vi "UDT_admittanceLibrary_InitialConditions FGV.vi"() -> (3 "Unit Test Framework Results":T1)   [LabVIEW 2017]
doc: "Use this template to create a user-defined test VI. Define your test requirements and wire the results to the <b>Result (Test)</b> control. Do not modify the <b>Unit Test Framework Results</b> indicator."
uses:
  <vilib>/utf/common/utf_test_result_troll.ctl
  <vilib>/utf/common/utf_test_result.ctl
  <vilib>/utf/common/utf_test_result_failure.ctl
  <vilib>/utf/common/utf_test_comparison_operators.ctl
  <vilib>/utf/common/utf_vi_tag.ctl
  RT/Admittance Controller/Controls/initial conditions control.ctl
  <vilib>/Control Software Solutions Ltd/UTF Helper/SubVIs/UTF Double Not Equals.vi
  <vilib>/Control Software Solutions Ltd/UTF Helper/SubVIs/UTF Double Equals.vi
  RT/Admittance Controller/admittanceControllerLibrary.lvlib
  <vilib>/Control Software Solutions Ltd/UTF Helper/Unit Test Helper.lvlib
  <vilib>/utf/NI_UnitTestFramework.lvlib
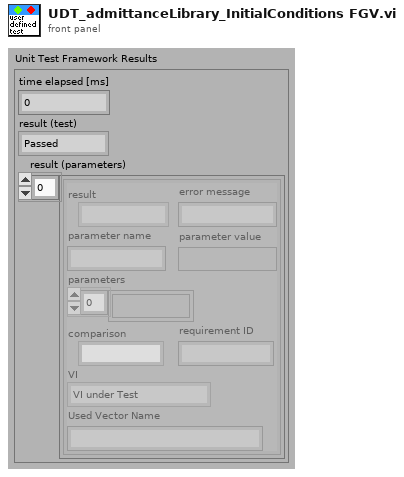
[diagram p1: front panel]
types:
  T1 = typedef "NI_UnitTestFramework.lvlib/utf_test_result_troll.ctl" = cluster{"time elapsed [ms]":u32, "result (test)":T2, "result (parameters)":T3[]}
  T2 = typedef "NI_UnitTestFramework.lvlib/utf_test_result.ctl" = enum16{"Passed", "Failed", "Error", "Skipped", "Not Processed"}
  T3 = typedef "NI_UnitTestFramework.lvlib/utf_test_result_failure.ctl" = cluster{"result":T2, "error message":string, "parameter name":string, "parameter value":variant, "parameters":variant[], "comparison":T4, "requirement ID":string, "VI":T5, "Used Vector Name":string}
  T4 = typedef "NI_UnitTestFramework.lvlib/utf_test_comparison_operators.ctl" = enum16{"=", "!=", ">", ">=", "<", "<=", "range", "symmetric tolerance", "asymmetric tolerance", "string contains", "string not contain", "array size", "string length", "array range", "by element", "array range (limit array)", "user-defined", "array contains", "array not contain", "vector length", "= (elm)", "!= (elm)", "= (case insensitive)", "!= (case insensitive)"}
  T5 = typedef "NI_UnitTestFramework.lvlib/utf_vi_tag.ctl" = enum16{"Setup VI", "VI under Test", "Teardown VI"}
  T6 = typedef "admittanceControllerLibrary.lvlib/initial conditions control.ctl" = enum16{"get", "set"}
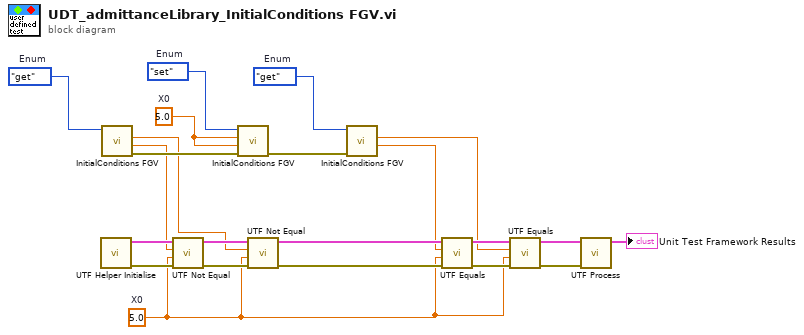
[diagram p0: block diagram]
diagram:
  w3 = 5.0  # X0
  w18 = initial_conditions_control."get"  # Enum
  w20 = initial_conditions_control."get"  # Enum
  w21 = 5.0  # X0
  w22 = initial_conditions_control."set"  # Enum
  n1 = call <vilib>:"UTF Helper Initialise.vi"() -> ("error out"=w14:errorcluster, "results array"=w15:T3[])  [unwired: 10 in]
  n2 = call "InitialConditions FGV.vi"("Enum"=w20) -> ("error out"=w19:errorcluster, "y0"=w11:dbl, "x0"=w10:dbl)  [unwired: 8 in]
  n3 = call-poly <vilib>:"UTF Not Equal.vi"("error in (no error)"=w14, "Test Value"=w3, "Input"=w11, "Input Results"=w15) -> ("error out"=w13:errorcluster, "Output Results"=w12:T3[])  [unwired: 6 in]
  n4 = call "InitialConditions FGV.vi"("error in (no error)"=w19, "Y0"=w21, "X0"=w21, "Enum"=w22) -> ("error out"=w17:errorcluster)  [unwired: 5 in, 2 out]
  n5 = call-poly <vilib>:"UTF Not Equal.vi"("error in (no error)"=w13, "Test Value"=w3, "Input"=w10, "Input Results"=w12) -> ("error out"=w8:errorcluster, "Output Results"=w9:T3[])  [unwired: 6 in]
  n6 = call "InitialConditions FGV.vi"("error in (no error)"=w17, "Enum"=w18) -> ("y0"=w5:dbl, "x0"=w4:dbl)  [unwired: 7 in, 1 out]
  n7 = call-poly <vilib>:"UTF Equals.vi"("error in (no error)"=w8, "Test Value"=w3, "Input"=w5, "Input Results"=w9) -> ("error out"=w6:errorcluster, "Output Results"=w7:T3[])  [unwired: 6 in]
  n8 = call-poly <vilib>:"UTF Equals.vi"("error in (no error)"=w6, "Test Value"=w3, "Input"=w4, "Input Results"=w7) -> ("error out"=w1:errorcluster, "Output Results"=w2:T3[])  [unwired: 6 in]
  n9 = call <vilib>:"UTF Process.vi"("error in (no error)"=w1, "results array"=w2) -> ("Unit Test Framework Results"=→"Unit Test Framework Results":T1)  [unwired: 9 in]
